vi "Python@GetVariable__Parameter.vi"(1 "ParamterIn":string) -> (0 "ParamterOut":string)   [LabVIEW 2019]
panel:
  in  "ARCOSName":string(combo) caption="ARCOSName="
  in  "Section":string(combo)
  in  "PythonVariable":string(combo)
  in  "Confirm":bool
  # "Python@GetVariable PythonVariable(,$section,ARCOSName=)"
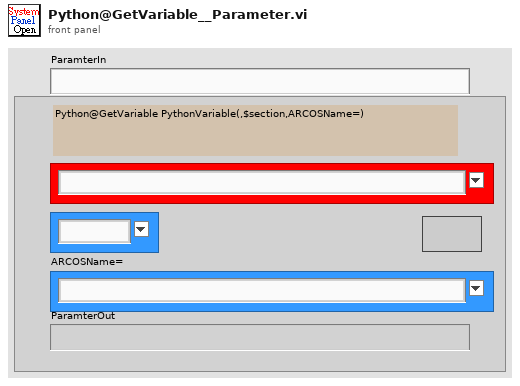
[diagram p1: front panel]
types:
  T1 = enum16{"Get", "Init", "Set", "Delete", "GetElement", "Inc", "Dec", "ReName"}
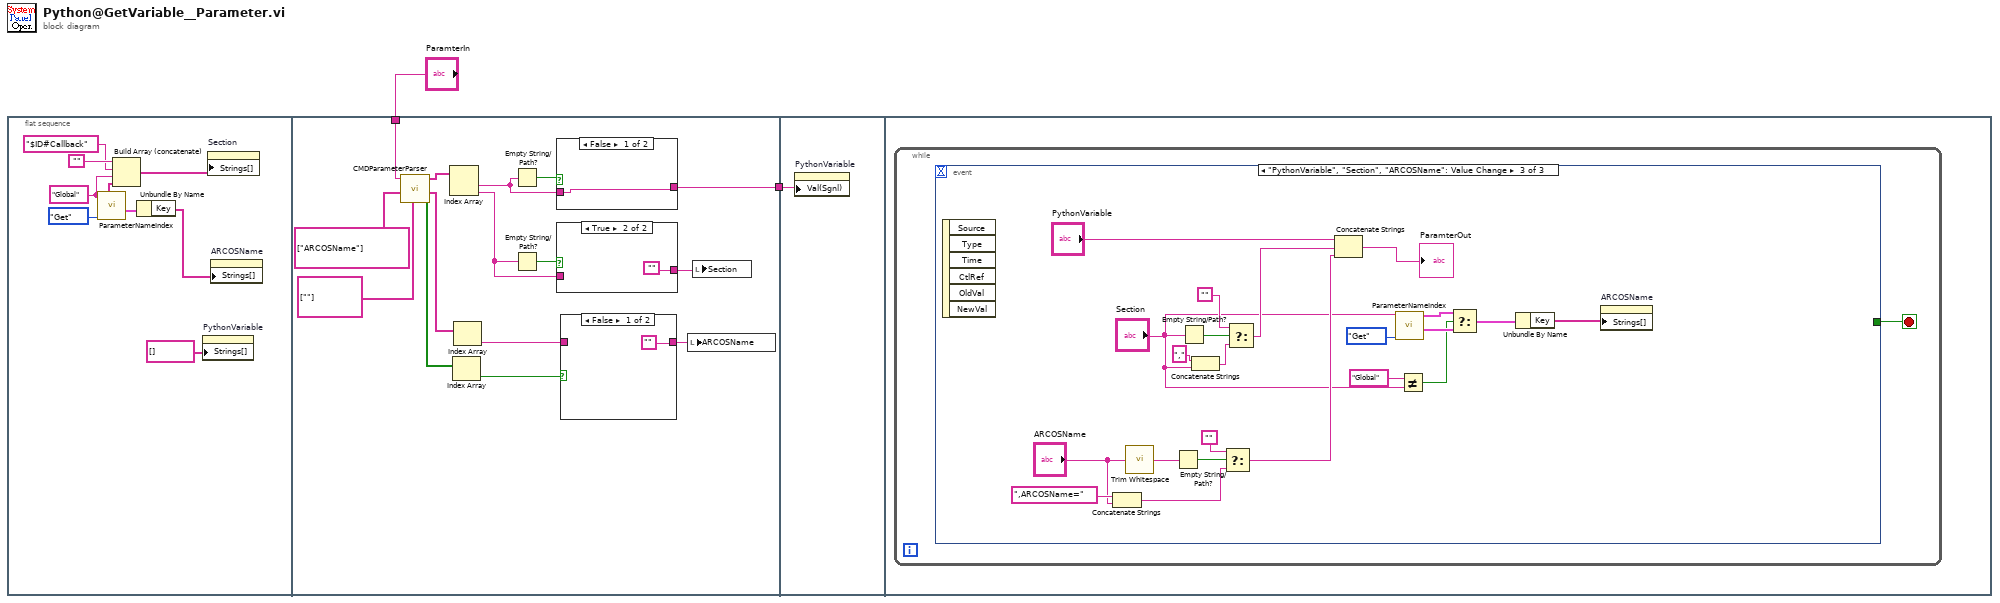
[diagram p0: block diagram]
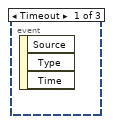
[diagram p5: hidden frame]
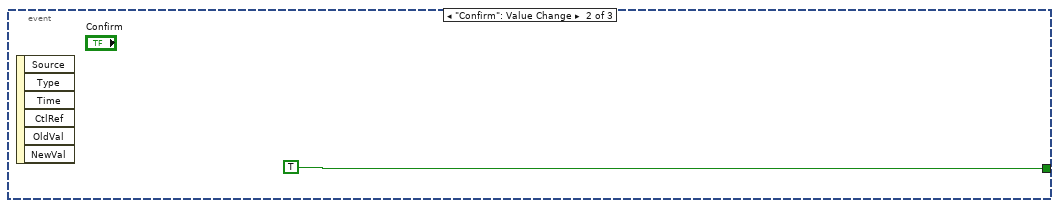
[diagram p6: hidden frame]
diagram:
  n1 = flat-sequence {
    tunnel: "ParamterIn" -> [w20]
    tunnel: [w25] -> w1
    tunnel: w1 -> [w33]
    frame #0 {
      w7 = "Global" ("VariableSection")
      n2 = call "ParameterNameIndex.vi"("OP"=T1."Get", "VariableSection"=w7) -> ("GlobalKeyValue"=w11:cluster{"Key":string[], "Value":string[]}, "SectionList"=w8:string[])  [unwired: 3 in, 5 out]
      n3 = Build Array (concatenate)("", "$ID#Callback" ("VariableSection"), w7, w8) -> (w6:string[])
      n4 = Unbundle By Name(w11) -> ("Key"=w4:string[])
      n5 = property on="PythonVariable" class="CmbBox"("Strings[]"=string[] [] ("Strings []")) -> ()  [unwired: 2 in, 2 out]
      n6 = property on="Section" class="CmbBox"("Strings[]"=w6) -> ()  [unwired: 2 in, 2 out]
      n7 = property on="ARCOSName" class="CmbBox"("Strings[]"=w4) -> ()  [unwired: 2 in, 2 out]
    }
    frame #1 {
      n8 = call "CMDParameterParser.vi"("DeafultValues"=string[] [""], "RequiredKeys"=string[] ["ARCOSName"], "CMDParameter"=w20) -> ("KeyFind?"=w15:bool[], "KeyValues"=w16:string[], "Input"=w19:string[])  [unwired: 6 in]
      n9 = Index Array(array=w19) -> (element #1=w24:string, element #2=w21:string)  [unwired: 2 in]
      n10 = Index Array(array=w15) -> (element=w14:bool)  [unwired: 1 in]
      n11 = Index Array(array=w16) -> (element=w13:string)  [unwired: 1 in]
      n12 = Empty String/Path?(string/path=w24) -> (empty?=w26:bool)
      n13 = Empty String/Path?(string/path=w21) -> (empty?=w23:bool)
      n14 = case shown="False" w26 {
        tunnel: w24 -> [w31 w32]
        tunnel: [w31 w32] -> w25
        frame False {
        }
        frame True {
        }
      }
      n15 = case shown="True" w23 {
        tunnel: w21 -> [w29 _]
        tunnel: [w29 ""] -> w22
        frame False {
        }
        frame True {
        }
      }
      n16 = case shown="False" w14 {
        tunnel: w13 -> [_ w28]
        tunnel: ["" w28] -> w12
        frame False {
        }
        frame True {
        }
      }
      n17 = local write "ARCOSName"(w12) -> ()
      n18 = local write "Section"(w22) -> ()
    }
    frame #2 {
      n19 = property on="PythonVariable" class="CmbBox"("Val(Sgnl)"=w33) -> ()  [unwired: 2 in, 2 out]
    }
    frame #3 {
      n20 = while {
        stop <- w34 stop-if-true
        n21 = event shown="[2] \"PythonVariable\", \"Section\", \"ARCOSName\": Value Change" {
          selector: _ -> [_ _ _]
          dyn-events: _ -> [_ _ _]
          timeout: _ -> [_ _ _]
          tunnel: [_ TRUE _] -> w34
          event Timeout {
            n22 = event-data() -> ()  [unwired: 1 in, 3 out]
          }
          event "Confirm": Value Change {
            n23 = event-data() -> ()  [unwired: 1 in, 6 out]
          }
          event "PythonVariable", "Section", "ARCOSName": Value Change {
            n24 = event-data() -> ()  [unwired: 1 in, 6 out]
            n25 = Concatenate Strings(",ARCOSName=" ("string"), "ARCOSName") -> (w43:string)
            n26 = call <vilib>:"Trim Whitespace.vi"("string"="ARCOSName") -> ("trimmed string"=w46:string)  [unwired: 1 in]
            n27 = Empty String/Path?(string/path=w46) -> (empty?=w45:bool)
            n28 = Empty String/Path?(string/path="Section") -> (empty?=w53:bool)
            n29 = Concatenate Strings("," ("string"), "Section") -> (w54:string)
            n30 = Select(t="", s=w45, f=w43) -> (s? t:f=w42:string)
            n31 = Select(t="", s=w53, f=w54) -> (s? t:f=w51:string)
            n32 = Concatenate Strings("PythonVariable", w51, w42) -> (→"ParamterOut":string)
            n33 = call "ParameterNameIndex.vi"("OP"=T1."Get", "VariableSection"="Section") -> ("GlobalKeyValue"=w40:cluster{"Key":string[], "Value":string[]}, "SectionKeyValue"=w41:cluster{"Key":string[], "Value":string[]})  [unwired: 3 in, 5 out]
            n34 = Not Equal?(x="Global", y="Section") -> (x != y?=w36:bool)
            n35 = Select(t=w41, s=w36, f=w40) -> (s? t:f=w39:cluster{"Key":string[], "Value":string[]})
            n36 = Unbundle By Name(w39) -> ("Key"=w49:string[])
            n37 = property on="ARCOSName" class="CmbBox"("Strings[]"=w49) -> ()  [unwired: 2 in, 2 out]
          }
        }
      }
    }
  }
